vi "Write On Count Status.vi"(8 "error in (no error)":errorcluster, 10 "On Count Status":T1, 11 "Repeat Until Count in":refnum<class "bt_Repeat Until Count.lvclass">) -> (0 "error out":errorcluster, 3 "Repeat Until Count out":refnum<class "bt_Repeat Until Count.lvclass">)   [LabVIEW 2021, in "BT.lvlib" / "bt_Repeat Until Count.lvclass"]
uses:
  bt_Repeat Until Count.lvclass
  Support/On Count Status - Type.ctl
  bt_Repeat Until Count.lvclass/bt_Repeat Until Count.ctl
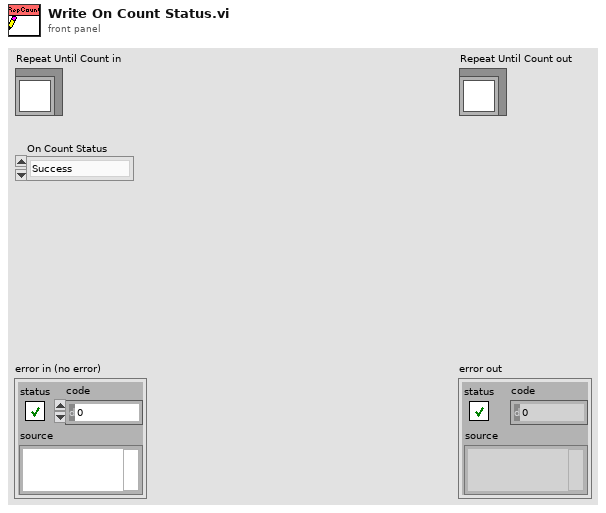
[diagram p1: front panel]
types:
  T1 = typedef "BT.lvlib/bt_Repeat Until Count.lvclass/On Count Status - Type.ctl" = enum16{"Success", "Failure"}
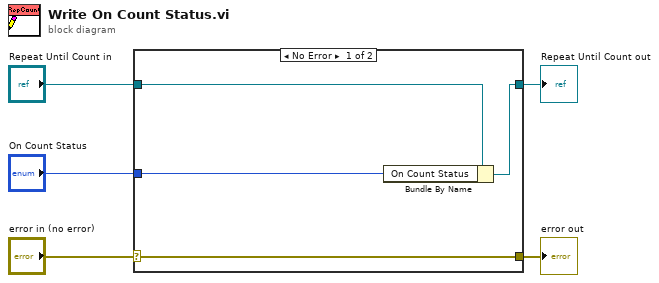
[diagram p0: block diagram]
diagram:
  n1 = case shown="No Error" "error in (no error)" {
    selector: "error in (no error)" -> [w9 w10]
    tunnel: [w9 w10] -> w4
    tunnel: [w7 w11] -> w2
    tunnel: "Repeat Until Count in" -> [w8 w11]
    tunnel: "On Count Status" -> [w6 _]
    frame No Error {
      n2 = Bundle By Name(cluster=w8, "On Count Status"=w6) -> (w7:refnum<class "bt_Repeat Until Count.lvclass">)
    }
    frame Error {
    }
  }
  "error out" <- w4
  "Repeat Until Count out" <- w2
